vi "writeDataFile.vi"(8 "error in (no error)":errorcluster, 10 "WriteDataFileInput":T1, 11 "CSVTestLog in":refnum<class "CSVTestLog.lvclass">) -> (0 "error out":errorcluster, 2 "Relative Path":string, 3 "CSVTestLog out":refnum<class "CSVTestLog.lvclass">)   [LabVIEW 2015, in "CSVTestLog.lvclass"]
uses:
  CSVTestLog.lvclass
  Typedefs/WriteDataFileInput.ctl
  CSVTestLog.lvclass/CSVTestLog.ctl
  Typedefs/FAMTTypedefs.lvlib
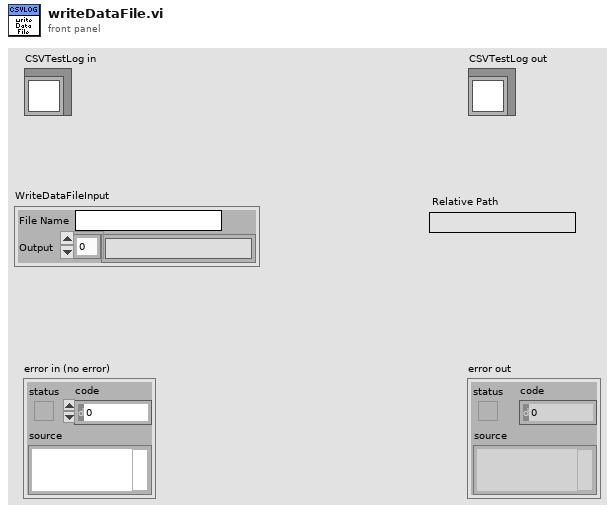
[diagram p1: front panel]
types:
  T1 = typedef "FAMTTypedefs.lvlib/WriteDataFileInput.ctl" = cluster{"File Name":string, "Output":string[]}
  T2 = enum16{"open", "replace", "create", "open or create", "replace or create", "replace or create with confirmation"}
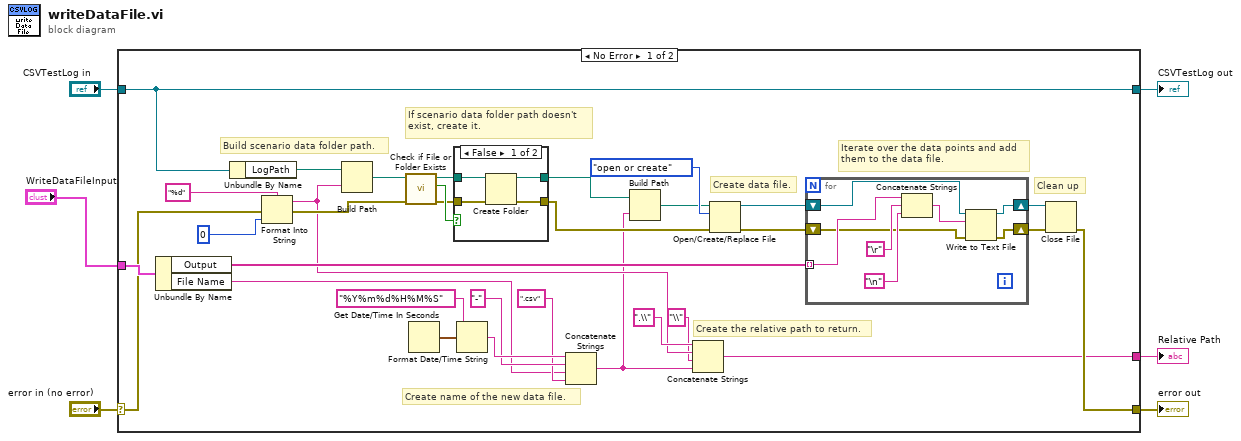
[diagram p0: block diagram]
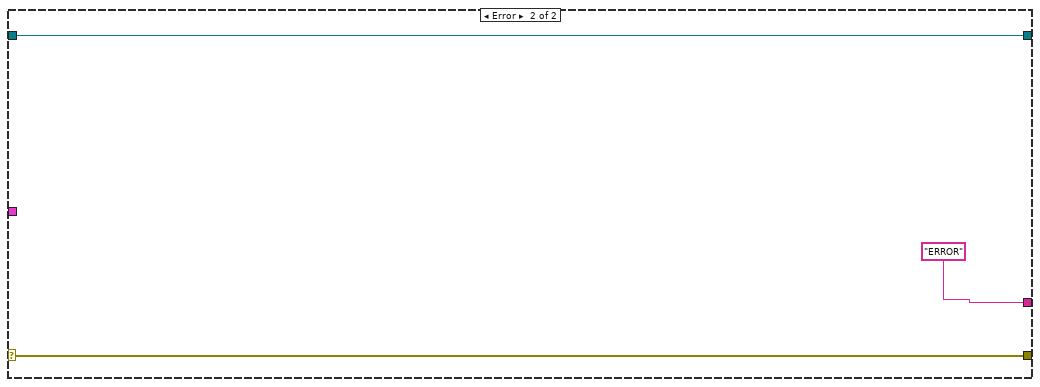
[diagram p3: hidden frame]
diagram:
  n1 = case shown="No Error" "error in (no error)" {
    selector: "error in (no error)" -> [w20 w55]
    tunnel: [w13 w55] -> w5
    tunnel: "CSVTestLog in" -> [w38 w54]
    tunnel: [w38 w54] -> w3
    tunnel: "WriteDataFileInput" -> [w32 _]
    tunnel: [w8 "ERROR"] -> w2
    frame No Error {
      # "Clean up"
      # "Iterate over the data points and add\nthem to the data file."
      # "Create data file."
      # "Create the relative path to return."
      # "Create name of the new data file."
      # "If scenario data folder path doesn't\nexist, create it."
      # "Build scenario data folder path."
      n2 = Unbundle By Name(w32) -> ("Output"=w18:string[], "File Name"=w19:string)
      n3 = Unbundle By Name(w38) -> ("LogPath"=w34:path)
      n4 = Format Into String(format string="%d", error in=w20, 0) -> (resulting string=w11:string, error out=w29:errorcluster)  [unwired: 1 in]
      n5 = Build Path(base path=w34, name or relative path=w11) -> (appended path=w33:path)
      n6 = call <vilib>:"Check if File or Folder Exists.vi"("error in (no error)"=w29, "path"=w33) -> ("error out"=w35:errorcluster, "file or folder exists?"=w37:bool, "dup path"=w36:path)  [unwired: 7 in]
      n7 = Get Date/Time In Seconds() -> (seconds since 1Jan1904=w26:timestamp)
      n8 = case shown="False" w37 {
        tunnel: w36 -> [w50 w52]
        tunnel: w35 -> [w49 w51]
        tunnel: [w48 w52] -> w30
        tunnel: [w47 w51] -> w22
        frame False {
          n9 = Create Folder(path (use dialog)=w50, error in=w49) -> (created path=w48:path, error out=w47:errorcluster)  [unwired: 1 in, 1 out]
        }
        frame True {
        }
      }
      n10 = Format Date/Time String(time format string (%c)="%Y%m%d%H%M%S", seconds (now)=w26) -> (date/time string=w28:string)  [unwired: 1 in]
      n11 = Concatenate Strings(w28, "-" ("string"), w19, ".csv" ("string")) -> (w9:string)
      n12 = Build Path(base path=w30, name or relative path=w9) -> (appended path=w21:path)
      n13 = Concatenate Strings(".\\" ("string"), w11, "\\" ("string"), w9) -> (w8:string)
      n14 = Open/Create/Replace File(file path (use dialog)=w21, error in=w22, operation (0:open)=T2."open or create") -> (refnum out=w17:refnum<file>, error out=w16:errorcluster)  [unwired: 3 in, 1 out]
      n15 = for {
        tunnel: w18 -> [w40] mode=indexing
        shift-right: [w42] -> w14
        shift-left: w16 -> [w39]
        shift-right: [w41] -> w15
        shift-left: w17 -> [w43]
        n16 = Concatenate Strings(w40, "\r", "\n") -> (w44:string)
        n17 = Write to Text File(file (use dialog)=w43, text=w44, error in=w39) -> (refnum out=w41:refnum<file>, error out=w42:errorcluster)  [unwired: 1 in, 1 out]
      }
      n18 = Close File(refnum=w15, error in=w14) -> (error out=w13:errorcluster)  [unwired: 1 out]
    }
    frame Error {
    }
  }
  "error out" <- w5
  "CSVTestLog out" <- w3
  "Relative Path" <- w2
